vi "Get 3-Byte Integer.vi"(11 "Bytes in":u8[](array[numeric])) -> (1 "3-Byte Integer":u64, 3 "Bytes out":u8[](array[numeric]))   [LabVIEW 2014, in "hse-db.lvlib" / "MySQL (TCP).lvlib"]
uses:
  MySQL (TCP).lvlib
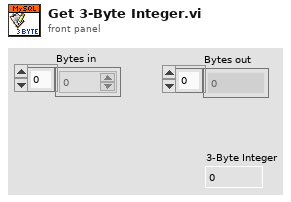
[diagram p1: front panel]
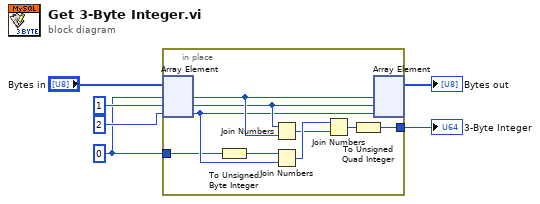
[diagram p0: block diagram]
diagram:
  w1 = 0
  n1 = in-place {
    in-place-border: [w15] -> w6
    in-place-border: w1 -> [w8]
    n2 = in-place-array #1("Bytes in", w1, 1, 2) -> (w11:u8, w10:u8, w9:u8)
    n3 = To Unsigned Byte Integer(number=w8) -> (unsigned 8bit integer=w7:u8)
    n4 = Join Numbers(hi=w10, lo=w11) -> ((hi.lo)=w12:u16)
    n5 = Join Numbers(hi=w7, lo=w9) -> ((hi.lo)=w13:u16)
    n6 = Join Numbers(hi=w13, lo=w12) -> ((hi.lo)=w14:u32)
    n7 = To Unsigned Quad Integer(1:w14) -> (0:w15:u64)
    n8 = in-place-array #1(w11, w10, w9) -> (→"Bytes out":u8[])  [unwired: 3 out]
  }
  "3-Byte Integer" <- w6
